vi "FGV SpanEinstellungen.vi"(5 "Punkte umkehren":bool[](array[boolean]) caption="Reverse points", 6 "Aktion":T13, 7 "PDF Optionen":T1, 8 "error in (no error)":errorcluster caption="Fehler (Eingang, kein Fehler)", 9 "automatisch in":T4, 10 "RegisterRefs":T3, 11 "SpanInletClusterArray in":T5[](array[typedef]) {"zusätzliche Zeitdauer Erster Punkt" min=30 step=1 format="%#_5g"; "Zeitdauer Stufen" format="%#_5g"; "Max Fehler" format="%#_5g"; "Anzahl Stufen" format="%#_5g"; "Komponenten"."Komponente 5"."Komponente:" items=["NO (350,3000) LP 191C", "NO2 (150) LP 191C (1of2)", "NO2 (2000) LP 191C (2of2)", "N2O (300) LP 191C (1of2)", "NH3 (300) LP 191C (1of2)", "NH3 (900,3000) LP 191C (2of2)", "HNCO (400) 191C", "H2O% (30) LP 191C", "Formaldehyde (70,500) LP 191C", "CO2 low% (4) LP 191C (2of2)", "CO2% (20) LP 191C (1of2)", "CO (700) LP 191C (1of3)", "CO% (1) LP 191C (2of3)", "Propylene (1000) LP 191C", "Aromatic HC C7 (500) LP 191C", "Ethylene (1000) LP 191C", "CH4 (250) LP 191C (1of2)", "CH4 (5000) LP 191C (2of2)", "Ethane (1000) LP 191C", "Acetylene (1000) LP 191C", "HNO2 (20) 191C", "MeOH (1000) 191C", "CO% (10) LP 191C (3of3)", "Formic Acid (100) 191C", "SO2 (500) LP 191C", "Acetaldehyde (1000) LP 191C", "COS (100) LP 191C", "1,3 butadiene (100) LP 191C", "Oil as Octane (200) LP 191C", "N2O (1000) LP 191C (2of2)", "Propane (200) LP 191C", "NO2 autorange (2000)", "CO autorange (100000)", "CH4 autorange (5000)", "NH3 autorange (3000)", "Temp. Gascell", "Pressure Gascell", "sBeam@2500"]; "Komponenten"."Komponente 5"."Konzentration IST" format="%#.4f"; "Komponenten"."Komponente 5"."Genauigkeit" format="%#.1f"; "Komponenten"."Komponente 4"."Komponente:" items=["NO (350,3000) LP 191C", "NO2 (150) LP 191C (1of2)", "NO2 (2000) LP 191C (2of2)", "N2O (300) LP 191C (1of2)", "NH3 (300) LP 191C (1of2)", "NH3 (900,3000) LP 191C (2of2)", "HNCO (400) 191C", "H2O% (30) LP 191C", "Formaldehyde (70,500) LP 191C", "CO2 low% (4) LP 191C (2of2)", "CO2% (20) LP 191C (1of2)", "CO (700) LP 191C (1of3)", "CO% (1) LP 191C (2of3)", "Propylene (1000) LP 191C", "Aromatic HC C7 (500) LP 191C", "Ethylene (1000) LP 191C", "CH4 (250) LP 191C (1of2)", "CH4 (5000) LP 191C (2of2)", "Ethane (1000) LP 191C", "Acetylene (1000) LP 191C", "HNO2 (20) 191C", "MeOH (1000) 191C", "CO% (10) LP 191C (3of3)", "Formic Acid (100) 191C", "SO2 (500) LP 191C", "Acetaldehyde (1000) LP 191C", "COS (100) LP 191C", "1,3 butadiene (100) LP 191C", "Oil as Octane (200) LP 191C", "N2O (1000) LP 191C (2of2)", "Propane (200) LP 191C", "NO2 autorange (2000)", "CO autorange (100000)", "CH4 autorange (5000)", "NH3 autorange (3000)", "Temp. Gascell", "Pressure Gascell", "sBeam@2500"]; "Komponenten"."Komponente 4"."Konzentration IST" format="%#.4f"; "Komponenten"."Komponente 4"."Genauigkeit" format="%#.1f"; "Komponenten"."Komponente 3"."Komponente:" items=["NO (350,3000) LP 191C", "NO2 (150) LP 191C (1of2)", "NO2 (2000) LP 191C (2of2)", "N2O (300) LP 191C (1of2)", "NH3 (300) LP 191C (1of2)", "NH3 (900,3000) LP 191C (2of2)", "HNCO (400) 191C", "H2O% (30) LP 191C", "Formaldehyde (70,500) LP 191C", "CO2 low% (4) LP 191C (2of2)", "CO2% (20) LP 191C (1of2)", "CO (700) LP 191C (1of3)", "CO% (1) LP 191C (2of3)", "Propylene (1000) LP 191C", "Aromatic HC C7 (500) LP 191C", "Ethylene (1000) LP 191C", "CH4 (250) LP 191C (1of2)", "CH4 (5000) LP 191C (2of2)", "Ethane (1000) LP 191C", "Acetylene (1000) LP 191C", "HNO2 (20) 191C", "MeOH (1000) 191C", "CO% (10) LP 191C (3of3)", "Formic Acid (100) 191C", "SO2 (500) LP 191C", "Acetaldehyde (1000) LP 191C", "COS (100) LP 191C", "1,3 butadiene (100) LP 191C", "Oil as Octane (200) LP 191C", "N2O (1000) LP 191C (2of2)", "Propane (200) LP 191C", "NO2 autorange (2000)", "CO autorange (100000)", "CH4 autorange (5000)", "NH3 autorange (3000)", "Temp. Gascell", "Pressure Gascell", "sBeam@2500"]; "Komponenten"."Komponente 3"."Konzentration IST" format="%#.4f"; "Komponenten"."Komponente 3"."Genauigkeit" format="%#.1f"; "Komponenten"."Komponente 2"."Komponente:" items=["NO (350,3000) LP 191C", "NO2 (150) LP 191C (1of2)", "NO2 (2000) LP 191C (2of2)", "N2O (300) LP 191C (1of2)", "NH3 (300) LP 191C (1of2)", "NH3 (900,3000) LP 191C (2of2)", "HNCO (400) 191C", "H2O% (30) LP 191C", "Formaldehyde (70,500) LP 191C", "CO2 low% (4) LP 191C (2of2)", "CO2% (20) LP 191C (1of2)", "CO (700) LP 191C (1of3)", "CO% (1) LP 191C (2of3)", "Propylene (1000) LP 191C", "Aromatic HC C7 (500) LP 191C", "Ethylene (1000) LP 191C", "CH4 (250) LP 191C (1of2)", "CH4 (5000) LP 191C (2of2)", "Ethane (1000) LP 191C", "Acetylene (1000) LP 191C", "HNO2 (20) 191C", "MeOH (1000) 191C", "CO% (10) LP 191C (3of3)", "Formic Acid (100) 191C", "SO2 (500) LP 191C", "Acetaldehyde (1000) LP 191C", "COS (100) LP 191C", "1,3 butadiene (100) LP 191C", "Oil as Octane (200) LP 191C", "N2O (1000) LP 191C (2of2)", "Propane (200) LP 191C", "NO2 autorange (2000)", "CO autorange (100000)", "CH4 autorange (5000)", "NH3 autorange (3000)", "Temp. Gascell", "Pressure Gascell", "sBeam@2500"]; "Komponenten"."Komponente 2"."Konzentration IST" format="%#.4f"; "Komponenten"."Komponente 2"."Genauigkeit" format="%#.1f"; "Komponenten"."Komponente 1"."Komponente:" items=["NO (350,3000) LP 191C", "NO2 (150) LP 191C (1of2)", "NO2 (2000) LP 191C (2of2)", "N2O (300) LP 191C (1of2)", "NH3 (300) LP 191C (1of2)", "NH3 (900,3000) LP 191C (2of2)", "HNCO (400) 191C", "H2O% (30) LP 191C", "Formaldehyde (70,500) LP 191C", "CO2 low% (4) LP 191C (2of2)", "CO2% (20) LP 191C (1of2)", "CO (700) LP 191C (1of3)", "CO% (1) LP 191C (2of3)", "Propylene (1000) LP 191C", "Aromatic HC C7 (500) LP 191C", "Ethylene (1000) LP 191C", "CH4 (250) LP 191C (1of2)", "CH4 (5000) LP 191C (2of2)", "Ethane (1000) LP 191C", "Acetylene (1000) LP 191C", "HNO2 (20) 191C", "MeOH (1000) 191C", "CO% (10) LP 191C (3of3)", "Formic Acid (100) 191C", "SO2 (500) LP 191C", "Acetaldehyde (1000) LP 191C", "COS (100) LP 191C", "1,3 butadiene (100) LP 191C", "Oil as Octane (200) LP 191C", "N2O (1000) LP 191C (2of2)", "Propane (200) LP 191C", "NO2 autorange (2000)", "CO autorange (100000)", "CH4 autorange (5000)", "NH3 autorange (3000)", "Temp. Gascell", "Pressure Gascell", "sBeam@2500"]; "Komponenten"."Komponente 1"."Konzentration IST" format="%#.4f"; "Komponenten"."Komponente 1"."Genauigkeit" format="%#.1f"; "Ablaufdatum" format="%<%d.%m.%Y>T"; "Gasflasche" items=["----"=10000, "IAG NH3 3000"=0, "IAG NH3 200"=1, "IAG NH3 2000"=2, "IAG MG"=3, "IAG O2"=4]}) -> (0 "error out":errorcluster caption="Fehler (Ausgang)", 1 "automatisch out":T4, 2 "RegisterRefs out":T3, 3 "SpanInletClusterArray out":T5[](array[typedef]) {"zusätzliche Zeitdauer Erster Punkt" min=30 step=1 format="%#_5g"; "Zeitdauer Stufen" format="%#_5g"; "Max Fehler" format="%#_5g"; "Anzahl Stufen" format="%#_5g"; "Komponenten"."Komponente 5"."Komponente:" items=["NO (350,3000) LP 191C", "NO2 (150) LP 191C (1of2)", "NO2 (2000) LP 191C (2of2)", "N2O (300) LP 191C (1of2)", "NH3 (300) LP 191C (1of2)", "NH3 (900,3000) LP 191C (2of2)", "HNCO (400) 191C", "H2O% (30) LP 191C", "Formaldehyde (70,500) LP 191C", "CO2 low% (4) LP 191C (2of2)", "CO2% (20) LP 191C (1of2)", "CO (700) LP 191C (1of3)", "CO% (1) LP 191C (2of3)", "Propylene (1000) LP 191C", "Aromatic HC C7 (500) LP 191C", "Ethylene (1000) LP 191C", "CH4 (250) LP 191C (1of2)", "CH4 (5000) LP 191C (2of2)", "Ethane (1000) LP 191C", "Acetylene (1000) LP 191C", "HNO2 (20) 191C", "MeOH (1000) 191C", "CO% (10) LP 191C (3of3)", "Formic Acid (100) 191C", "SO2 (500) LP 191C", "Acetaldehyde (1000) LP 191C", "COS (100) LP 191C", "1,3 butadiene (100) LP 191C", "Oil as Octane (200) LP 191C", "N2O (1000) LP 191C (2of2)", "Propane (200) LP 191C", "NO2 autorange (2000)", "CO autorange (100000)", "CH4 autorange (5000)", "NH3 autorange (3000)", "Temp. Gascell", "Pressure Gascell", "sBeam@2500"]; "Komponenten"."Komponente 5"."Konzentration IST" format="%#.4f"; "Komponenten"."Komponente 5"."Genauigkeit" format="%#.1f"; "Komponenten"."Komponente 4"."Komponente:" items=["NO (350,3000) LP 191C", "NO2 (150) LP 191C (1of2)", "NO2 (2000) LP 191C (2of2)", "N2O (300) LP 191C (1of2)", "NH3 (300) LP 191C (1of2)", "NH3 (900,3000) LP 191C (2of2)", "HNCO (400) 191C", "H2O% (30) LP 191C", "Formaldehyde (70,500) LP 191C", "CO2 low% (4) LP 191C (2of2)", "CO2% (20) LP 191C (1of2)", "CO (700) LP 191C (1of3)", "CO% (1) LP 191C (2of3)", "Propylene (1000) LP 191C", "Aromatic HC C7 (500) LP 191C", "Ethylene (1000) LP 191C", "CH4 (250) LP 191C (1of2)", "CH4 (5000) LP 191C (2of2)", "Ethane (1000) LP 191C", "Acetylene (1000) LP 191C", "HNO2 (20) 191C", "MeOH (1000) 191C", "CO% (10) LP 191C (3of3)", "Formic Acid (100) 191C", "SO2 (500) LP 191C", "Acetaldehyde (1000) LP 191C", "COS (100) LP 191C", "1,3 butadiene (100) LP 191C", "Oil as Octane (200) LP 191C", "N2O (1000) LP 191C (2of2)", "Propane (200) LP 191C", "NO2 autorange (2000)", "CO autorange (100000)", "CH4 autorange (5000)", "NH3 autorange (3000)", "Temp. Gascell", "Pressure Gascell", "sBeam@2500"]; "Komponenten"."Komponente 4"."Konzentration IST" format="%#.4f"; "Komponenten"."Komponente 4"."Genauigkeit" format="%#.1f"; "Komponenten"."Komponente 3"."Komponente:" items=["NO (350,3000) LP 191C", "NO2 (150) LP 191C (1of2)", "NO2 (2000) LP 191C (2of2)", "N2O (300) LP 191C (1of2)", "NH3 (300) LP 191C (1of2)", "NH3 (900,3000) LP 191C (2of2)", "HNCO (400) 191C", "H2O% (30) LP 191C", "Formaldehyde (70,500) LP 191C", "CO2 low% (4) LP 191C (2of2)", "CO2% (20) LP 191C (1of2)", "CO (700) LP 191C (1of3)", "CO% (1) LP 191C (2of3)", "Propylene (1000) LP 191C", "Aromatic HC C7 (500) LP 191C", "Ethylene (1000) LP 191C", "CH4 (250) LP 191C (1of2)", "CH4 (5000) LP 191C (2of2)", "Ethane (1000) LP 191C", "Acetylene (1000) LP 191C", "HNO2 (20) 191C", "MeOH (1000) 191C", "CO% (10) LP 191C (3of3)", "Formic Acid (100) 191C", "SO2 (500) LP 191C", "Acetaldehyde (1000) LP 191C", "COS (100) LP 191C", "1,3 butadiene (100) LP 191C", "Oil as Octane (200) LP 191C", "N2O (1000) LP 191C (2of2)", "Propane (200) LP 191C", "NO2 autorange (2000)", "CO autorange (100000)", "CH4 autorange (5000)", "NH3 autorange (3000)", "Temp. Gascell", "Pressure Gascell", "sBeam@2500"]; "Komponenten"."Komponente 3"."Konzentration IST" format="%#.4f"; "Komponenten"."Komponente 3"."Genauigkeit" format="%#.1f"; "Komponenten"."Komponente 2"."Komponente:" items=["NO (350,3000) LP 191C", "NO2 (150) LP 191C (1of2)", "NO2 (2000) LP 191C (2of2)", "N2O (300) LP 191C (1of2)", "NH3 (300) LP 191C (1of2)", "NH3 (900,3000) LP 191C (2of2)", "HNCO (400) 191C", "H2O% (30) LP 191C", "Formaldehyde (70,500) LP 191C", "CO2 low% (4) LP 191C (2of2)", "CO2% (20) LP 191C (1of2)", "CO (700) LP 191C (1of3)", "CO% (1) LP 191C (2of3)", "Propylene (1000) LP 191C", "Aromatic HC C7 (500) LP 191C", "Ethylene (1000) LP 191C", "CH4 (250) LP 191C (1of2)", "CH4 (5000) LP 191C (2of2)", "Ethane (1000) LP 191C", "Acetylene (1000) LP 191C", "HNO2 (20) 191C", "MeOH (1000) 191C", "CO% (10) LP 191C (3of3)", "Formic Acid (100) 191C", "SO2 (500) LP 191C", "Acetaldehyde (1000) LP 191C", "COS (100) LP 191C", "1,3 butadiene (100) LP 191C", "Oil as Octane (200) LP 191C", "N2O (1000) LP 191C (2of2)", "Propane (200) LP 191C", "NO2 autorange (2000)", "CO autorange (100000)", "CH4 autorange (5000)", "NH3 autorange (3000)", "Temp. Gascell", "Pressure Gascell", "sBeam@2500"]; "Komponenten"."Komponente 2"."Konzentration IST" format="%#.4f"; "Komponenten"."Komponente 2"."Genauigkeit" format="%#.1f"; "Komponenten"."Komponente 1"."Komponente:" items=["NO (350,3000) LP 191C", "NO2 (150) LP 191C (1of2)", "NO2 (2000) LP 191C (2of2)", "N2O (300) LP 191C (1of2)", "NH3 (300) LP 191C (1of2)", "NH3 (900,3000) LP 191C (2of2)", "HNCO (400) 191C", "H2O% (30) LP 191C", "Formaldehyde (70,500) LP 191C", "CO2 low% (4) LP 191C (2of2)", "CO2% (20) LP 191C (1of2)", "CO (700) LP 191C (1of3)", "CO% (1) LP 191C (2of3)", "Propylene (1000) LP 191C", "Aromatic HC C7 (500) LP 191C", "Ethylene (1000) LP 191C", "CH4 (250) LP 191C (1of2)", "CH4 (5000) LP 191C (2of2)", "Ethane (1000) LP 191C", "Acetylene (1000) LP 191C", "HNO2 (20) 191C", "MeOH (1000) 191C", "CO% (10) LP 191C (3of3)", "Formic Acid (100) 191C", "SO2 (500) LP 191C", "Acetaldehyde (1000) LP 191C", "COS (100) LP 191C", "1,3 butadiene (100) LP 191C", "Oil as Octane (200) LP 191C", "N2O (1000) LP 191C (2of2)", "Propane (200) LP 191C", "NO2 autorange (2000)", "CO autorange (100000)", "CH4 autorange (5000)", "NH3 autorange (3000)", "Temp. Gascell", "Pressure Gascell", "sBeam@2500"]; "Komponenten"."Komponente 1"."Konzentration IST" format="%#.4f"; "Komponenten"."Komponente 1"."Genauigkeit" format="%#.1f"; "Ablaufdatum" format="%<%d.%m.%Y>T"; "Gasflasche" items=["----"=10000, "IAG NH3 3000"=0, "IAG NH3 200"=1, "IAG NH3 2000"=2, "IAG MG"=3, "IAG O2"=4]}, 4 "Punkte umkehren und PDF Optionen Cluster":T2)   [LabVIEW 2020, in "Linearisierung v2.lvlib" / "SpanEinstellungen.lvlib"]
uses:
  SpanEinstellungen.lvlib
  Aktion FGV SpanEinstellungen.ctl
  SpanInletCluster.ctl
  Seiten/System Einstellungen V2/Konfig Gasflasche.ctl
  Seiten/System Einstellungen V2/Analysatoren.ctl
  Seiten/System Einstellungen V2/Gasflasche Auswahl.ctl
  Komponentencluster mit Formel.ctl
  Komponentenauswahl mit Formel.ctl
  Visualisierungs Elemente/String - Eingabefeld.ctl
  Einheit.ctl
  Seiten/System Einstellungen V2/Traegergas.ctl
  PDF Optionen.ctl
  Allgemein/allgemeine Sub-VIs.lvlib
  Seiten/System Einstellungen V2/System Einstellungen V2.lvlib
panel:
  # "sec"
  # "%"
  # "sec"
  # "Komponente"
  # "Formel"
  # "Konzentration"
  # "Einheit"
  # "Genauigkeit [%]"
  # "sec"
  # "%"
  # "sec"
  # "Komponente"
  # "Formel"
  # "Konzentration"
  # "Einheit"
  # "Genauigkeit [%]"
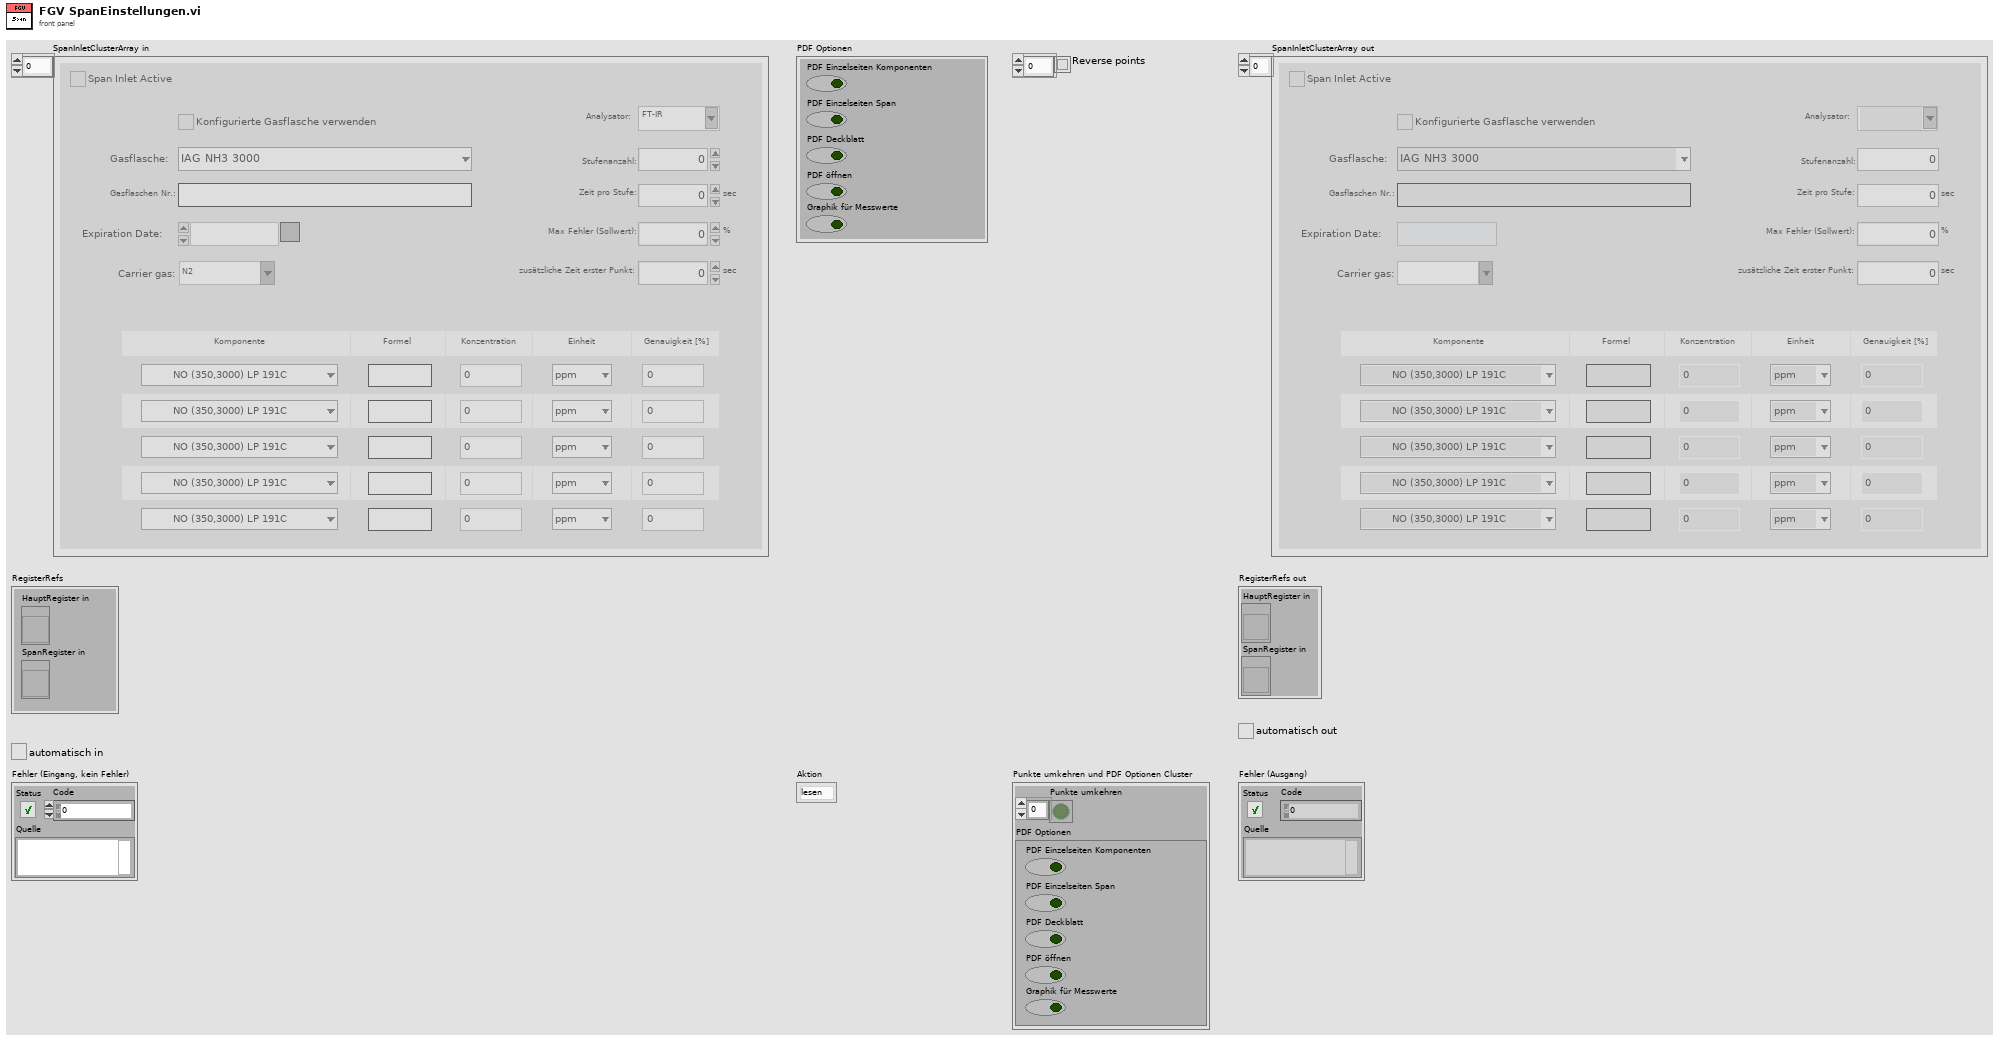
[diagram p1: front panel]
types:
  T1 = typedef "Linearisierung v2.lvlib/SpanEinstellungen.lvlib/PDF Optionen.ctl" = cluster{"PDF Einzelseiten Komponenten":bool, "PDF Einzelseiten Span":bool, "PDF Deckblatt":bool, "PDF öffnen":bool, "Graphik für Messwerte":bool}
  T2 = cluster{"Punkte umkehren":bool[], "PDF Optionen":T1}
  T3 = cluster{"HauptRegister in":refnum<vi>, "SpanRegister in":refnum<vi>}
  T4 = typedef "System Einstellungen V2.lvlib/Konfig Gasflasche.ctl" = bool
  T5 = typedef "Linearisierung v2.lvlib/SpanEinstellungen.lvlib/SpanInletCluster.ctl" = cluster{"Span Inlet Active":T4, "Analysator":T6, "Konfig Gasflasche":T4, "Gasflasche":T7, "Gasflaschen Nr.:":string, "Ablaufdatum":timestamp, "Komponenten":T8, "Zeitdauer Stufen":sgl, "Max Fehler":sgl, "Anzahl Stufen":sgl, "Trägergas":T12, "zusätzliche Zeitdauer Erster Punkt":sgl}
  T6 = typedef "System Einstellungen V2.lvlib/Analysatoren.ctl" = string
  T7 = typedef "System Einstellungen V2.lvlib/Gasflasche Auswahl.ctl" = u16
  T8 = typedef "Linearisierung v2.lvlib/SpanEinstellungen.lvlib/Komponentencluster mit Formel.ctl" = cluster{"Komponente 1":T9, "Komponente 2":T9, "Komponente 3":T9, "Komponente 4":T9, "Komponente 5":T9}
  T9 = typedef "Linearisierung v2.lvlib/SpanEinstellungen.lvlib/Komponentenauswahl mit Formel.ctl" = cluster{"Komponente:":u16, "Summenformel":T10, "Konzentration IST":dbl, "Einheit":T11, "Genauigkeit":dbl}
  T10 = typedef "String - Eingabefeld.ctl" = string
  T11 = typedef "Linearisierung v2.lvlib/SpanEinstellungen.lvlib/Einheit.ctl" = enum16{"ppm", "%"}
  T12 = typedef "System Einstellungen V2.lvlib/Traegergas.ctl" = string
  T13 = typedef "Linearisierung v2.lvlib/SpanEinstellungen.lvlib/Aktion FGV SpanEinstellungen.ctl" = enum16{"lesen", "schreiben", "laden", "speichern", "RegisterRef", "automatisch", "init", "PDF Params", "Punkte umkehren"}
  T14 = enum16{"open", "replace", "create", "open or create", "replace or create", "replace or create with confirmation"}
  T15 = cluster{"automatisch in":T4, "SpanInletClusterArray in":T5[], "Punkte umkehren":bool[], "PDF Optionen":T1}
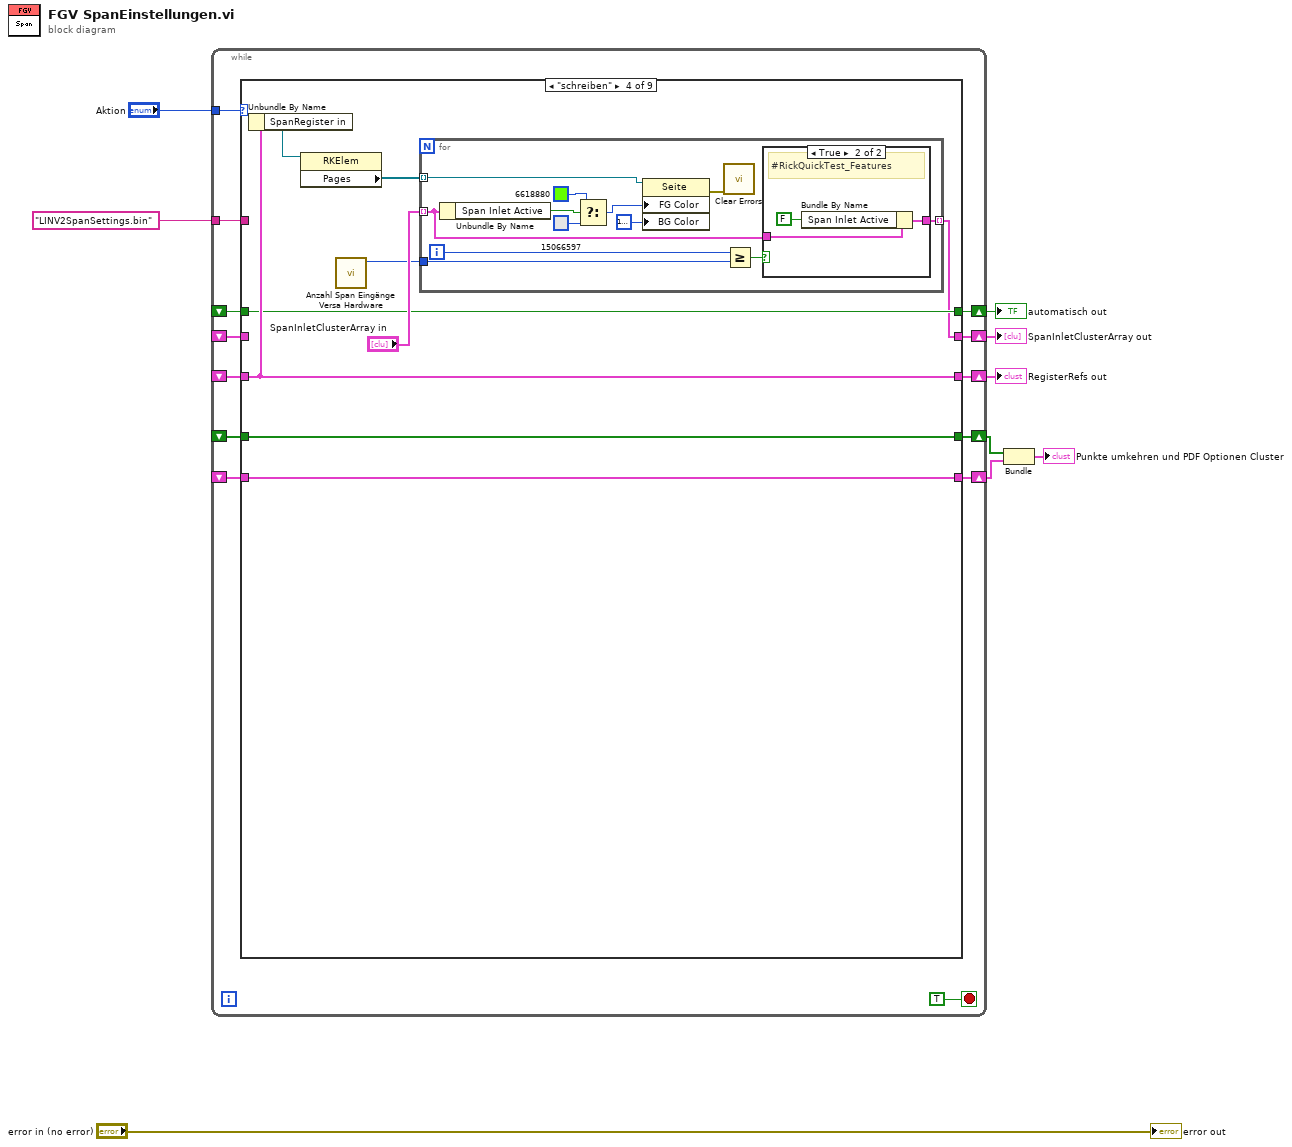
[diagram p0: block diagram]
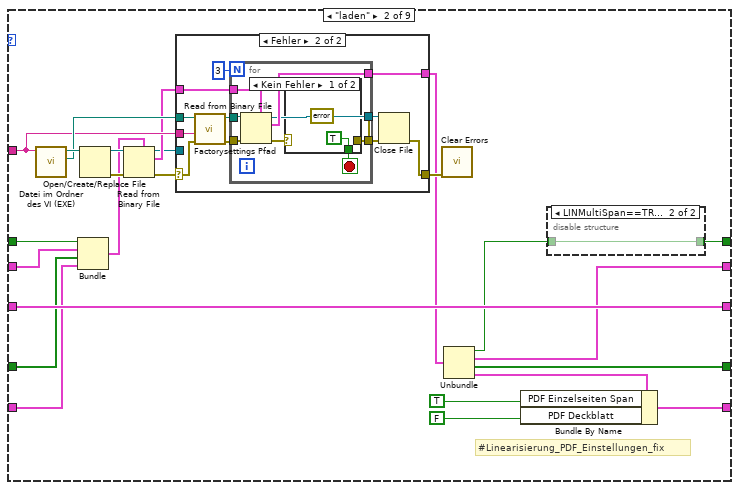
[diagram p3: hidden frame]
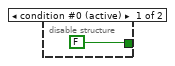
[diagram p4: hidden frame]
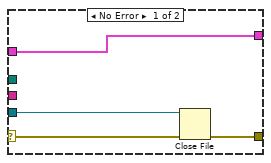
[diagram p5: hidden frame]
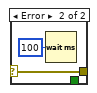
[diagram p6: hidden frame]
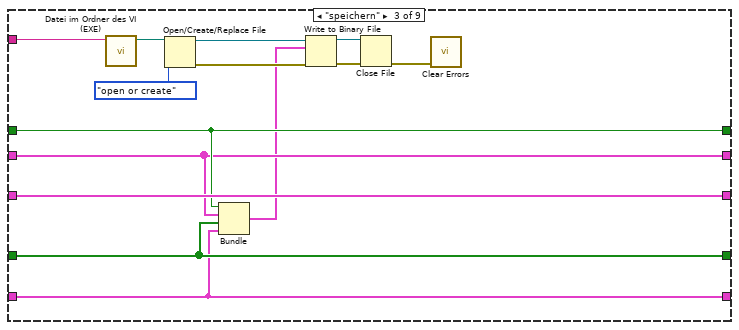
[diagram p7: hidden frame]
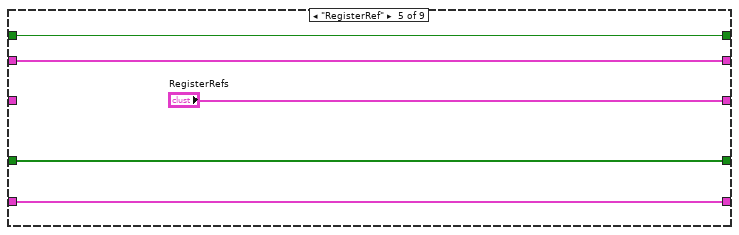
[diagram p9: hidden frame]
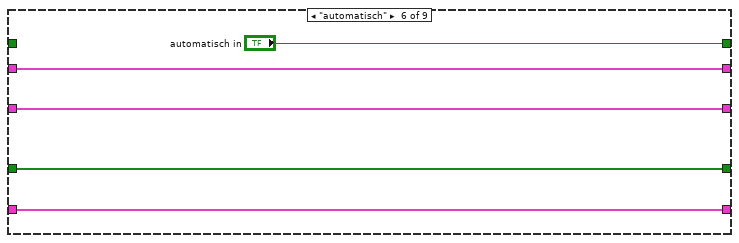
[diagram p10: hidden frame]
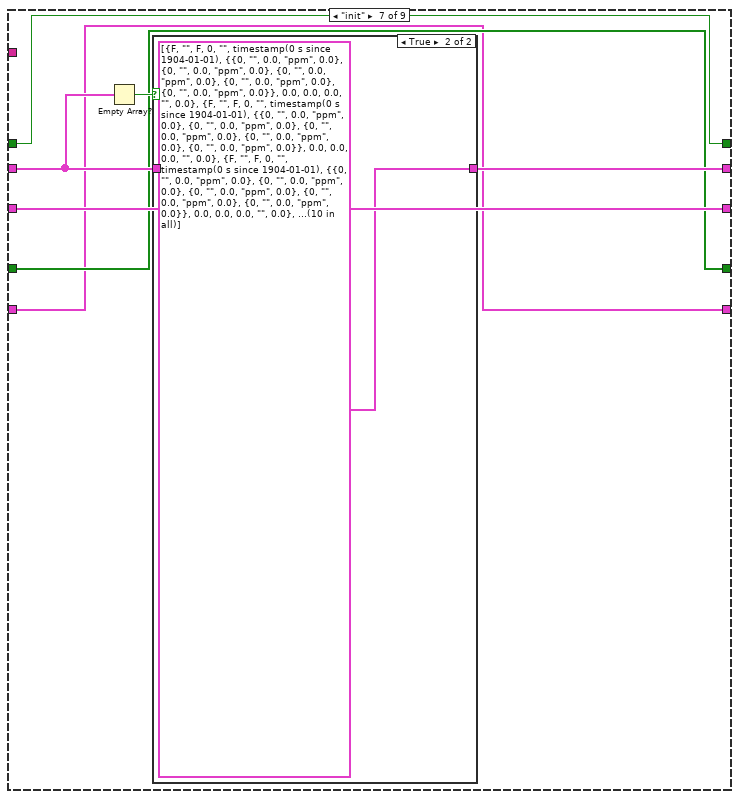
[diagram p11: hidden frame]
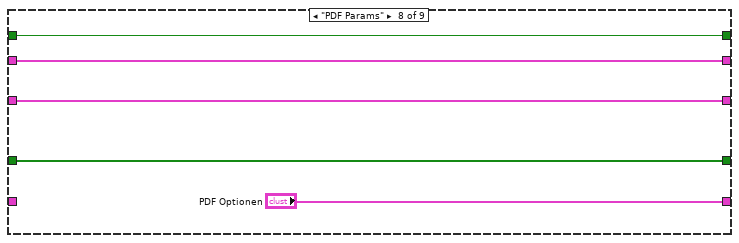
[diagram p13: hidden frame]
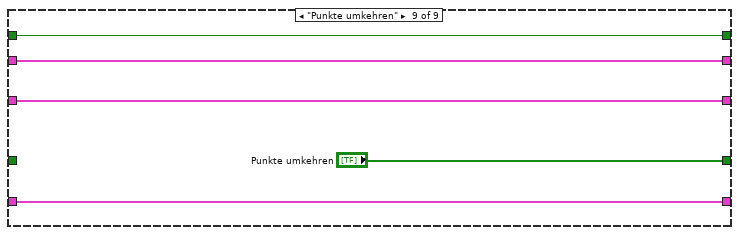
[diagram p14: hidden frame]
diagram:
  n1 = while {
    tunnel: "Aktion" -> [w21]
    tunnel: "LINV2SpanSettings.bin" ("Dateiname") -> [w20]
    shift-right: [w19] -> w7
    shift-left: _ -> [w18]
    shift-right: [w17] -> w5
    shift-left: _ -> [w16]
    shift-right: [w15] -> w4
    shift-left: _ -> [w14]
    shift-right: [w13] -> w3
    shift-left: _ -> [w12]
    shift-right: [w11] -> w2
    shift-left: _ -> [w10]
    stop <- TRUE stop-if-true
    n2 = case shown="\"schreiben\"" w21 {
      tunnel: w20 -> [_ w47 w87 _ _ _ _ _ _]
      tunnel: [w27 w37 w84 w95 w124 w129 w133 w143 w148] -> w19
      tunnel: w18 -> [w27 w40 w84 _ w124 w129 w134 w143 w148]
      tunnel: [w26 w42 w86 w103 "RegisterRefs" w128 w136 w142 w147] -> w17
      tunnel: w16 -> [w26 w42 w86 w103 _ w128 w136 w142 w147]
      tunnel: [w25 w32 w85 w100 w123 "automatisch in" w132 w141 w146] -> w15
      tunnel: w14 -> [w25 w41 w85 w100 w123 _ w132 w141 w146]
      tunnel: [w24 w35 w82 w98 w121 w126 w131 w140 "Punkte umkehren"] -> w13
      tunnel: w12 -> [w24 w36 w82 w98 w121 w126 w131 w140 _]
      tunnel: [w23 w28 w81 w97 w120 w125 w130 "PDF Optionen" w144] -> w11
      tunnel: w10 -> [w23 w34 w81 w97 w120 w125 w130 _ w144]
      frame "lesen", Default {
      }
      frame "laden" {
        # "#Linearisierung_PDF_Einstellungen_fix"
        n3 = call "Datei im Ordner des VI (EXE).vi"("Dateiname"=w47) -> ("Ordner des Haupt-VIs"=w48:path, "Dateipfad im Ordner des Haupt-VIs"=w51:path)  [unwired: 8 in, 1 out]
        n4 = Bundle("automatisch in"=w41, "SpanInletClusterArray in"=w40, "Punkte umkehren"=w36, "PDF Optionen"=w34) -> (w39:T15)  [unwired: 1 in]
        n5 = Open/Create/Replace File(file path (use dialog)=w51) -> (refnum out=w49:refnum<file>, error out=w50:errorcluster)  [unwired: 5 in, 1 out]
        n6 = Read from Binary File(5:w39, 8:w50, 11:w49) -> (0:w46:errorcluster, 2:w45:T15, 3:w43:refnum<file>)  [unwired: 3 in, 1 out]
        n7 = case shown="Fehler" w46 {
          selector: w46 -> [w56 w60]
          tunnel: w48 -> [_ w61]
          tunnel: w45 -> [w57 w59]
          tunnel: [w57 w67] -> w38
          tunnel: [w54 w65] -> w44
          tunnel: w43 -> [w55 _]
          tunnel: w47 -> [_ w58]
          frame No Error {
            n8 = Close File(refnum=w55, error in=w56) -> (error out=w54:errorcluster)  [unwired: 1 out]
          }
          frame Error {
            n9 = call "Factorysettings Pfad.vi"("error in (no error)"=w60, "Dateiname"=w58, "Ordner des Haupt-VIs"=w61) -> ("error out"=w62:errorcluster, "Pfad Factorysettings"=w63:path)  [unwired: 7 in]
            n10 = for {
              N: 3 -> [_]
              tunnel: w62 -> [w74]
              tunnel: w63 -> [w73]
              tunnel: [w72] -> w67
              tunnel: [w71] -> w66
              tunnel: [w70] -> w64
              tunnel: w59 -> [w69]
              stop <- w75 stop-if-true
              n11 = Read from Binary File(5:w69, 8:w74, 11:w73) -> (0:w76:errorcluster, 2:w72:T15, 3:w70:refnum<file>)  [unwired: 3 in, 1 out]
              n12 = case shown="Kein Fehler" w76 {
                selector: w76 -> [_ w79]
                tunnel: [TRUE _] -> w75
                tunnel: [errorcluster {"status"=FALSE, "code"=0, "source"=""} ("error IO") w79] -> w71
                frame No Error {
                }
                frame Error {
                  n13 = Wait (ms)(milliseconds to wait=u32 100 ("Zu wartende ms")) -> ()  [unwired: 1 out]
                }
              }
            }
            n14 = Close File(refnum=w64, error in=w66) -> (error out=w65:errorcluster)  [unwired: 1 out]
          }
        }
        n15 = call <vilib>:"Clear Errors.vi"("error in (no error)"=w44) -> ()  [unwired: 5 in, 2 out]
        n16 = Unbundle(w38) -> ("automatisch in"=w33:T4, "SpanInletClusterArray in"=w37:T5[], "Punkte umkehren"=w35:bool[], "PDF Optionen"=w31:T1)
        n17 = Bundle By Name(cluster=w31, "PDF Einzelseiten Span"=TRUE ("PDF Einzelseiten"), "PDF Deckblatt"=FALSE) -> (w28:T1)
        n18 = disable-structure shown="LINMultiSpan==TRUE" {
          disable-tunnel: w33 -> [_ w53]
          disable-tunnel: [FALSE w53] -> w32
          frame condition #0 (active) {
          }
          frame condition #1 {
          }
        }
      }
      frame "speichern" {
        n19 = call "Datei im Ordner des VI (EXE).vi"("Dateiname"=w87) -> ("Dateipfad im Ordner des Haupt-VIs"=w93:path)  [unwired: 8 in, 2 out]
        n20 = Open/Create/Replace File(file path (use dialog)=w93, operation (0:open)=T14."open or create" ("Operation (0:open)")) -> (refnum out=w92:refnum<file>, error out=w94:errorcluster)  [unwired: 4 in, 1 out]
        n21 = Bundle("automatisch in"=w85, "SpanInletClusterArray in"=w84, "Punkte umkehren"=w82, "PDF Optionen"=w81) -> (w83:T15)  [unwired: 1 in]
        n22 = Write to Binary File(file (use dialog)=w92, data=w83, error in=w94) -> (refnum out=w91:refnum<file>, error out=w90:errorcluster)  [unwired: 3 in, 1 out]
        n23 = Close File(refnum=w91, error in=w90) -> (error out=w89:errorcluster)  [unwired: 1 out]
        n24 = call <vilib>:"Clear Errors.vi"("error in (no error)"=w89) -> ()  [unwired: 5 in, 2 out]
      }
      frame "schreiben" {
        n25 = Unbundle By Name(w103) -> ("SpanRegister in"=w99:refnum<vi>)
        n26 = property class="RKElem"(reference=w99) -> ("Pages"=w102:refnum<vi>[])  [unwired: 1 in, 2 out]
        n27 = call "Anzahl Span Eingänge Versa Hardware.vi"() -> ("Anzahl Span"=w96:i32)  [unwired: 11 in]
        n28 = for {
          tunnel: "SpanInletClusterArray in" -> [w105] mode=indexing
          tunnel: w102 -> [w109] mode=indexing
          tunnel: w96 -> [w107]
          tunnel: [w104] -> w95 mode=indexing
          i -> [w108]
          n29 = Unbundle By Name(w105) -> ("Span Inlet Active"=w110:T4)
          n30 = Select(t=u32 6618880, s=w110, f=u32 15066597) -> (s? t:f=w114:u32)
          n31 = property class="Seite"(reference=w109, "FG Color"=w114, "BG Color"=u32 16777226) -> (error out=w115:errorcluster)  [unwired: 1 in, 1 out]
          n32 = call <vilib>:"Clear Errors.vi"("error in (no error)"=w115) -> ()  [unwired: 5 in, 2 out]
          n33 = Greater Or Equal?(x=w108, y=w107) -> (x >= y?=w106:bool)
          n34 = case shown="True" w106 {
            tunnel: w105 -> [w116 w119]
            tunnel: [w116 w117] -> w104
            frame False {
            }
            frame True {
              # "#RickQuickTest_Features"
              n35 = Bundle By Name(cluster=w119, "Span Inlet Active"=T4 FALSE) -> (w117:T5)
            }
          }
        }
      }
      frame "RegisterRef" {
      }
      frame "automatisch" {
      }
      frame "init" {
        n36 = Empty Array?(array=w134) -> (empty?=w135:bool)
        n37 = case shown="True" w135 {
          tunnel: w134 -> [w137 _]
          tunnel: [w137 T5[] [{"Span Inlet Active"=FALSE, "Analysator"="", "Konfig Gasflasche"=FALSE, "Gasflasche"=0, "Gasflaschen Nr.:"="", "Ablaufdatum"=timestamp(0 s since 1904-01-01), "Komponenten"={"Komponente 1"={"Komponente:"=0, "Summenformel"="", "Konzentration IST"=0.0, "Einheit"=enum."ppm", "Genauigkeit"=0.0}, "Komponente 2"={"Komponente:"=0, "Summenformel"="", "Konzentration IST"=0.0, "Einheit"=enum."ppm", "Genauigkeit"=0.0}, "Komponente 3"={"Komponente:"=0, "Summenformel"="", "Konzentration IST"=0.0, "Einheit"=enum."ppm", "Genauigkeit"=0.0}, "Komponente 4"={"Komponente:"=0, "Summenformel"="", "Konzentration IST"=0.0, "Einheit"=enum."ppm", "Genauigkeit"=0.0}, "Komponente 5"={"Komponente:"=0, "Summenformel"="", "Konzentration IST"=0.0, "Einheit"=enum."ppm", "Genauigkeit"=0.0}}, "Zeitdauer Stufen"=0.0, "Max Fehler"=0.0, "Anzahl Stufen"=0.0, "Trägergas"="", "zusätzliche Zeitdauer Erster Punkt"=0.0}, {"Span Inlet Active"=FALSE, "Analysator"="", "Konfig Gasflasche"=FALSE, "Gasflasche"=0, "Gasflaschen Nr.:"="", "Ablaufdatum"=timestamp(0 s since 1904-01-01), "Komponenten"={"Komponente 1"={"Komponente:"=0, "Summenformel"="", "Konzentration IST"=0.0, "Einheit"=enum."ppm", "Genauigkeit"=0.0}, "Komponente 2"={"Komponente:"=0, "Summenformel"="", "Konzentration IST"=0.0, "Einheit"=enum."ppm", "Genauigkeit"=0.0}, "Komponente 3"={"Komponente:"=0, "Summenformel"="", "Konzentration IST"=0.0, "Einheit"=enum."ppm", "Genauigkeit"=0.0}, "Komponente 4"={"Komponente:"=0, "Summenformel"="", "Konzentration IST"=0.0, "Einheit"=enum."ppm", "Genauigkeit"=0.0}, "Komponente 5"={"Komponente:"=0, "Summenformel"="", "Konzentration IST"=0.0, "Einheit"=enum."ppm", "Genauigkeit"=0.0}}, "Zeitdauer Stufen"=0.0, "Max Fehler"=0.0, "Anzahl Stufen"=0.0, "Trägergas"="", "zusätzliche Zeitdauer Erster Punkt"=0.0}, {"Span Inlet Active"=FALSE, "Analysator"="", "Konfig Gasflasche"=FALSE, "Gasflasche"=0, "Gasflaschen Nr.:"="", "Ablaufdatum"=timestamp(0 s since 1904-01-01), "Komponenten"={"Komponente 1"={"Komponente:"=0, "Summenformel"="", "Konzentration IST"=0.0, "Einheit"=enum."ppm", "Genauigkeit"=0.0}, "Komponente 2"={"Komponente:"=0, "Summenformel"="", "Konzentration IST"=0.0, "Einheit"=enum."ppm", "Genauigkeit"=0.0}, "Komponente 3"={"Komponente:"=0, "Summenformel"="", "Konzentration IST"=0.0, "Einheit"=enum."ppm", "Genauigkeit"=0.0}, "Komponente 4"={"Komponente:"=0, "Summenformel"="", "Konzentration IST"=0.0, "Einheit"=enum."ppm", "Genauigkeit"=0.0}, "Komponente 5"={"Komponente:"=0, "Summenformel"="", "Konzentration IST"=0.0, "Einheit"=enum."ppm", "Genauigkeit"=0.0}}, "Zeitdauer Stufen"=0.0, "Max Fehler"=0.0, "Anzahl Stufen"=0.0, "Trägergas"="", "zusätzliche Zeitdauer Erster Punkt"=0.0}, {"Span Inlet Active"=FALSE, "Analysator"="", "Konfig Gasflasche"=FALSE, "Gasflasche"=0, "Gasflaschen Nr.:"="", "Ablaufdatum"=timestamp(0 s since 1904-01-01), "Komponenten"={"Komponente 1"={"Komponente:"=0, "Summenformel"="", "Konzentration IST"=0.0, "Einheit"=enum."ppm", "Genauigkeit"=0.0}, "Komponente 2"={"Komponente:"=0, "Summenformel"="", "Konzentration IST"=0.0, "Einheit"=enum."ppm", "Genauigkeit"=0.0}, "Komponente 3"={"Komponente:"=0, "Summenformel"="", "Konzentration IST"=0.0, "Einheit"=enum."ppm", "Genauigkeit"=0.0}, "Komponente 4"={"Komponente:"=0, "Summenformel"="", "Konzentration IST"=0.0, "Einheit"=enum."ppm", "Genauigkeit"=0.0}, "Komponente 5"={"Komponente:"=0, "Summenformel"="", "Konzentration IST"=0.0, "Einheit"=enum."ppm", "Genauigkeit"=0.0}}, "Zeitdauer Stufen"=0.0, "Max Fehler"=0.0, "Anzahl Stufen"=0.0, "Trägergas"="", "zusätzliche Zeitdauer Erster Punkt"=0.0}, {"Span Inlet Active"=FALSE, "Analysator"="", "Konfig Gasflasche"=FALSE, "Gasflasche"=0, "Gasflaschen Nr.:"="", "Ablaufdatum"=timestamp(0 s since 1904-01-01), "Komponenten"={"Komponente 1"={"Komponente:"=0, "Summenformel"="", "Konzentration IST"=0.0, "Einheit"=enum."ppm", "Genauigkeit"=0.0}, "Komponente 2"={"Komponente:"=0, "Summenformel"="", "Konzentration IST"=0.0, "Einheit"=enum."ppm", "Genauigkeit"=0.0}, "Komponente 3"={"Komponente:"=0, "Summenformel"="", "Konzentration IST"=0.0, "Einheit"=enum."ppm", "Genauigkeit"=0.0}, "Komponente 4"={"Komponente:"=0, "Summenformel"="", "Konzentration IST"=0.0, "Einheit"=enum."ppm", "Genauigkeit"=0.0}, "Komponente 5"={"Komponente:"=0, "Summenformel"="", "Konzentration IST"=0.0, "Einheit"=enum."ppm", "Genauigkeit"=0.0}}, "Zeitdauer Stufen"=0.0, "Max Fehler"=0.0, "Anzahl Stufen"=0.0, "Trägergas"="", "zusätzliche Zeitdauer Erster Punkt"=0.0}, {"Span Inlet Active"=FALSE, "Analysator"="", "Konfig Gasflasche"=FALSE, "Gasflasche"=0, "Gasflaschen Nr.:"="", "Ablaufdatum"=timestamp(0 s since 1904-01-01), "Komponenten"={"Komponente 1"={"Komponente:"=0, "Summenformel"="", "Konzentration IST"=0.0, "Einheit"=enum."ppm", "Genauigkeit"=0.0}, "Komponente 2"={"Komponente:"=0, "Summenformel"="", "Konzentration IST"=0.0, "Einheit"=enum."ppm", "Genauigkeit"=0.0}, "Komponente 3"={"Komponente:"=0, "Summenformel"="", "Konzentration IST"=0.0, "Einheit"=enum."ppm", "Genauigkeit"=0.0}, "Komponente 4"={"Komponente:"=0, "Summenformel"="", "Konzentration IST"=0.0, "Einheit"=enum."ppm", "Genauigkeit"=0.0}, "Komponente 5"={"Komponente:"=0, "Summenformel"="", "Konzentration IST"=0.0, "Einheit"=enum."ppm", "Genauigkeit"=0.0}}, "Zeitdauer Stufen"=0.0, "Max Fehler"=0.0, "Anzahl Stufen"=0.0, "Trägergas"="", "zusätzliche Zeitdauer Erster Punkt"=0.0}, {"Span Inlet Active"=FALSE, "Analysator"="", "Konfig Gasflasche"=FALSE, "Gasflasche"=0, "Gasflaschen Nr.:"="", "Ablaufdatum"=timestamp(0 s since 1904-01-01), "Komponenten"={"Komponente 1"={"Komponente:"=0, "Summenformel"="", "Konzentration IST"=0.0, "Einheit"=enum."ppm", "Genauigkeit"=0.0}, "Komponente 2"={"Komponente:"=0, "Summenformel"="", "Konzentration IST"=0.0, "Einheit"=enum."ppm", "Genauigkeit"=0.0}, "Komponente 3"={"Komponente:"=0, "Summenformel"="", "Konzentration IST"=0.0, "Einheit"=enum."ppm", "Genauigkeit"=0.0}, "Komponente 4"={"Komponente:"=0, "Summenformel"="", "Konzentration IST"=0.0, "Einheit"=enum."ppm", "Genauigkeit"=0.0}, "Komponente 5"={"Komponente:"=0, "Summenformel"="", "Konzentration IST"=0.0, "Einheit"=enum."ppm", "Genauigkeit"=0.0}}, "Zeitdauer Stufen"=0.0, "Max Fehler"=0.0, "Anzahl Stufen"=0.0, "Trägergas"="", "zusätzliche Zeitdauer Erster Punkt"=0.0}, {"Span Inlet Active"=FALSE, "Analysator"="", "Konfig Gasflasche"=FALSE, "Gasflasche"=0, "Gasflaschen Nr.:"="", "Ablaufdatum"=timestamp(0 s since 1904-01-01), "Komponenten"={"Komponente 1"={"Komponente:"=0, "Summenformel"="", "Konzentration IST"=0.0, "Einheit"=enum."ppm", "Genauigkeit"=0.0}, "Komponente 2"={"Komponente:"=0, "Summenformel"="", "Konzentration IST"=0.0, "Einheit"=enum."ppm", "Genauigkeit"=0.0}, "Komponente 3"={"Komponente:"=0, "Summenformel"="", "Konzentration IST"=0.0, "Einheit"=enum."ppm", "Genauigkeit"=0.0}, "Komponente 4"={"Komponente:"=0, "Summenformel"="", "Konzentration IST"=0.0, "Einheit"=enum."ppm", "Genauigkeit"=0.0}, "Komponente 5"={"Komponente:"=0, "Summenformel"="", "Konzentration IST"=0.0, "Einheit"=enum."ppm", "Genauigkeit"=0.0}}, "Zeitdauer Stufen"=0.0, "Max Fehler"=0.0, "Anzahl Stufen"=0.0, "Trägergas"="", "zusätzliche Zeitdauer Erster Punkt"=0.0}, {"Span Inlet Active"=FALSE, "Analysator"="", "Konfig Gasflasche"=FALSE, "Gasflasche"=0, "Gasflaschen Nr.:"="", "Ablaufdatum"=timestamp(0 s since 1904-01-01), "Komponenten"={"Komponente 1"={"Komponente:"=0, "Summenformel"="", "Konzentration IST"=0.0, "Einheit"=enum."ppm", "Genauigkeit"=0.0}, "Komponente 2"={"Komponente:"=0, "Summenformel"="", "Konzentration IST"=0.0, "Einheit"=enum."ppm", "Genauigkeit"=0.0}, "Komponente 3"={"Komponente:"=0, "Summenformel"="", "Konzentration IST"=0.0, "Einheit"=enum."ppm", "Genauigkeit"=0.0}, "Komponente 4"={"Komponente:"=0, "Summenformel"="", "Konzentration IST"=0.0, "Einheit"=enum."ppm", "Genauigkeit"=0.0}, "Komponente 5"={"Komponente:"=0, "Summenformel"="", "Konzentration IST"=0.0, "Einheit"=enum."ppm", "Genauigkeit"=0.0}}, "Zeitdauer Stufen"=0.0, "Max Fehler"=0.0, "Anzahl Stufen"=0.0, "Trägergas"="", "zusätzliche Zeitdauer Erster Punkt"=0.0}, {"Span Inlet Active"=FALSE, "Analysator"="", "Konfig Gasflasche"=FALSE, "Gasflasche"=0, "Gasflaschen Nr.:"="", "Ablaufdatum"=timestamp(0 s since 1904-01-01), "Komponenten"={"Komponente 1"={"Komponente:"=0, "Summenformel"="", "Konzentration IST"=0.0, "Einheit"=enum."ppm", "Genauigkeit"=0.0}, "Komponente 2"={"Komponente:"=0, "Summenformel"="", "Konzentration IST"=0.0, "Einheit"=enum."ppm", "Genauigkeit"=0.0}, "Komponente 3"={"Komponente:"=0, "Summenformel"="", "Konzentration IST"=0.0, "Einheit"=enum."ppm", "Genauigkeit"=0.0}, "Komponente 4"={"Komponente:"=0, "Summenformel"="", "Konzentration IST"=0.0, "Einheit"=enum."ppm", "Genauigkeit"=0.0}, "Komponente 5"={"Komponente:"=0, "Summenformel"="", "Konzentration IST"=0.0, "Einheit"=enum."ppm", "Genauigkeit"=0.0}}, "Zeitdauer Stufen"=0.0, "Max Fehler"=0.0, "Anzahl Stufen"=0.0, "Trägergas"="", "zusätzliche Zeitdauer Erster Punkt"=0.0}] ("SpanInletClusterArray in")] -> w133
          frame False {
          }
          frame True {
          }
        }
      }
      frame "PDF Params" {
      }
      frame "Punkte umkehren" {
      }
    }
  }
  "SpanInletClusterArray out" <- w7
  "automatisch out" <- w4
  "RegisterRefs out" <- w5
  n38 = Bundle("Punkte umkehren"=w3, "PDF Optionen"=w2) -> (→"Punkte umkehren und PDF Optionen Cluster":T2)  [unwired: 1 in]
  "error out" <- "error in (no error)"
